vi "Measurement Logic.vi"(8 "error in":errorcluster, 9 "measurement configuration":T2={"Automation Test"=FALSE, "Power sequencing file path"="", "RFSG name"="5842_0", "RFSG port"="", "RFSG attenuation mode"=enum."Constant Attenuation", "RFSG external attenuation (dB)"=2.0, "RFSG s-parameters orientation"=enum."Port2 Towards DUT", "RFSG s2p file path"="", "RFmx name"="5842_0", "RFmx port"="", "RFmx attenuation mode"=enum."Constant Attenuation", "RFmx external attenuation (dB)"=1.2, "RFmx s-parameters orientation"=enum."Port2 Towards DUT", "RFmx s2p file path"="", "RFmx Center Frequency (Hz)"=10000000000.0, "RFmx Measurement Bandwidth (Hz)"=80000000.0, "RFmx Reference Level (dBm)"=10.0, "RFSG Generation IQ Rate (S/s)"=10000000000.0, "Pulse Acquisition Length (s)"=80000000.0, "Pulse Power Level (dBm)"=10.0, "Pulse Repetition Interval [PRI] (s)"=1250000000.0, "Pulse Width (s)"=0.001, "Number of Pulses per Burst"=0, "Measurement Offset"=0, "Window Start (%)"=2e-05, "Window Stop (%)"=20.0, "Window Step Size (%)"=0.0, "High Reference Level (%)"=10.0, "Width Reference Level (%)"=90.0, "Low Reference Level (%)"=10.0, "Selected Pulse Trace"=0, "Power sequencing file validity check"=FALSE} {"Width Reference Level (%)" format="%.2p"; "Window Stop (%)" format="%#_6p"; "Window Start (%)" format="%#_6p"; "Measurement Offset" format="%#_6p"; "Pulse Acquisition Length (s)" format="%.2f"; "Pulse Power Level (dBm)" format="%.6p"; "Number of Pulses per Burst" format="%.2f"; "Pulse Width (s)" format="%.3p"; "Pulse Repetition Interval [PRI] (s)" format="%.6p"; "RFSG Generation IQ Rate (S/s)" format="%.3p"; "RFmx Reference Level (dBm)" format="%.6p"; "RFmx Measurement Bandwidth (Hz)" format="%.3p"; "RFmx Center Frequency (Hz)" format="%.6p"; "RFmx external attenuation (dB)" format="%.2f"; "RFSG external attenuation (dB)" format="%.2f"}, 10 "measure call context in":refnum<class "Measure Call Context.lvclass">) -> (0 "error out":errorcluster, 1 "measurement results":T1, 2 "measure call context out":refnum<class "Measure Call Context.lvclass">)   [LabVIEW 2023, in "FPT Pulse Measurement.lvclass"]
doc: "Contains the core logic for executing the measurement."
uses:
  FPT Pulse Measurement.lvclass
  <vilib>/Plug-In SDKs/Measurements/Measure Call Context/Measure Call Context.lvclass
  Measurement Configuration.ctl
  Measurement Results.ctl
  <vilib>/Analysis/baseanly.llb/Mean (DBL).vi
  <extravilib>/ChannelInstances/Event Messenger-bool/Instantiate.vi
  FPT Pulse Measurement.lvclass/FPT Pulse Measurement.ctl
  <vilib>/Analysis/NI_AALBase.lvlib
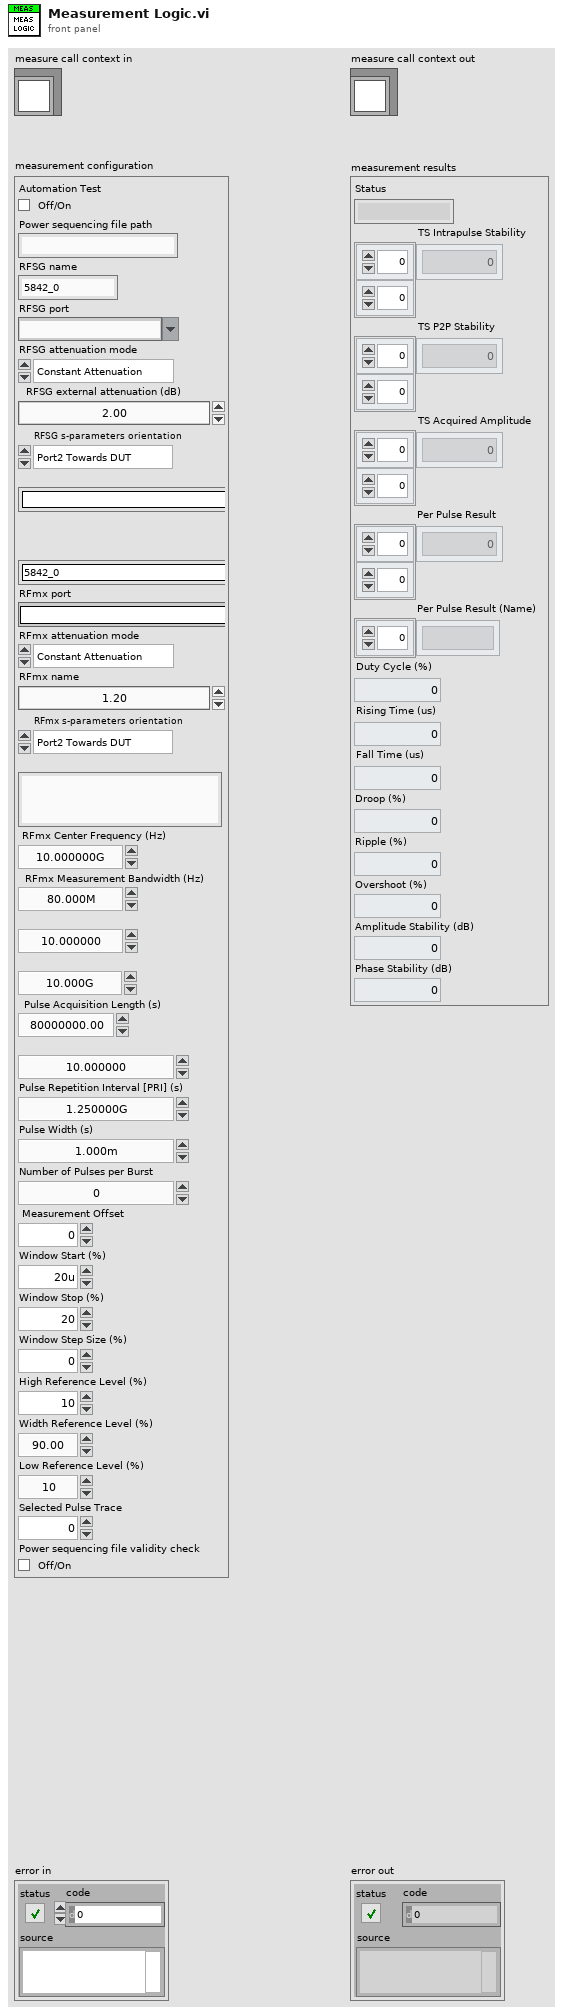
[diagram p1: front panel]
types:
  T1 = typedef "FPT Pulse Measurement.lvclass/Measurement Results.ctl" = cluster{"Status":string, "TS Intrapulse Stability":dbl[][], "TS P2P Stability":dbl[][], "TS Acquired Amplitude":dbl[][], "Per Pulse Result":dbl[][], "Per Pulse Result (Name)":string[], "Duty Cycle (%)":dbl, "Rising Time (us)":dbl, "Fall Time (us)":dbl, "Droop (%)":dbl, "Ripple (%)":dbl, "Overshoot (%)":dbl, "Amplitude Stability (dB)":dbl, "Phase Stability (dB)":dbl}
  T2 = typedef "FPT Pulse Measurement.lvclass/Measurement Configuration.ctl" = cluster{"Automation Test":bool, "Power sequencing file path":string, "RFSG name":string, "RFSG port":string, "RFSG attenuation mode":enum32{"<None>", "Constant Attenuation", "s2p File"}, "RFSG external attenuation (dB)":dbl, "RFSG s-parameters orientation":enum32{"Port1 Towards DUT", "Port2 Towards DUT"}, "RFSG s2p file path":string, "RFmx name":string, "RFmx port":string, "RFmx attenuation mode":enum32{"<None>", "Constant Attenuation", "s2p File"}, "RFmx external attenuation (dB)":dbl, "RFmx s-parameters orientation":enum32{"Port1 Towards DUT", "Port2 Towards DUT"}, "RFmx s2p file path":string, "RFmx Center Frequency (Hz)":dbl, "RFmx Measurement Bandwidth (Hz)":dbl, "RFmx Reference Level (dBm)":dbl, "RFSG Generation IQ Rate (S/s)":dbl, "Pulse Acquisition Length (s)":dbl, "Pulse Power Level (dBm)":dbl, "Pulse Repetition Interval [PRI] (s)":dbl, "Pulse Width (s)":dbl, "Number of Pulses per Burst":u32, "Measurement Offset":i32, "Window Start (%)":dbl, "Window Stop (%)":dbl, "Window Step Size (%)":dbl, "High Reference Level (%)":dbl, "Width Reference Level (%)":dbl, "Low Reference Level (%)":dbl, "Selected Pulse Trace":i32, "Power sequencing file validity check":bool}
  T3 = enum32{"Power On Dut", "De-embedding + Measurement", "Power Off Dut"}[]
  T4 = cluster{"measurement configuration":T2, "measurement results":T1, "CustomData":cluster{"Valid CSV":bool}}
  T5 = typedef "RFmx Config - Pulse.ctl" = cluster{"Center Frequency (Hz)":dbl, "Measurement Bandwidth (Hz)":dbl, "Reference Level (dBm)":dbl, "RFmx De-embedding":T6, "Acquisition Length (s)":dbl}
  T6 = typedef "RFmx Config.ctl" = cluster{"RFmx Name":refnum<k15>, "RFmx Port":string, "Attenuation":cluster{"Mode":enum32{"<None>", "Constant Attenuation", "s2p File"}, "Constant Attenuation":cluster{"RFmx External Attenuation (dB)":dbl}, "s2p File":cluster{"RFmx S-Parameters Orientation":i32, "RFmx Attenuation s2p Path Name":string, "RFmx Attenuation s2p File":path}}}
  T7 = typedef "RFSG Config - Pulse.ctl" = cluster{"RFSG De-embedding":T8, "Generation IQ Rate (S/s)":dbl}
  T8 = typedef "RFsg Config.ctl" = cluster{"RFSG Name":refnum<k15>, "RFSG Port":string, "Attenuation":cluster{"Mode":enum32{"<None>", "Constant Attenuation", "s2p File"}, "Contant Attenuation":cluster{"RFSG External Attenuation (dB)":dbl}, "s2p File":cluster{"RFSG S-parameters Orientation":i32, "RFSG Attenuation s2p Path Name":string, "RFSG s2p File Path":path}}}
  T9 = typedef "Test Config - Pulse.ctl" = cluster{"Pulse Configuration":cluster{"Power Level (dBm)":dbl, "Pulse Repetition Interval [PRI] (s)":dbl, "Pulse Width (s)":dbl, "Number of Pulses per Burst":u32}, "Pulse Stability":cluster{"Pulse Stability Meas Offset":i32, "Window Start (%)":dbl, "Window Stop (%)":dbl, "Window Step Size (%)":dbl, "Selected Pulse Trace":i32}, "Pulse Profile":cluster{"High Reference Level (%)":dbl, "Width Reference Level (%)":dbl, "Low Reference Level (%)":dbl}}
  T10 = typedef "Event Messenger-bool.lvlib/))Channel.ctl" = refnum<queue>
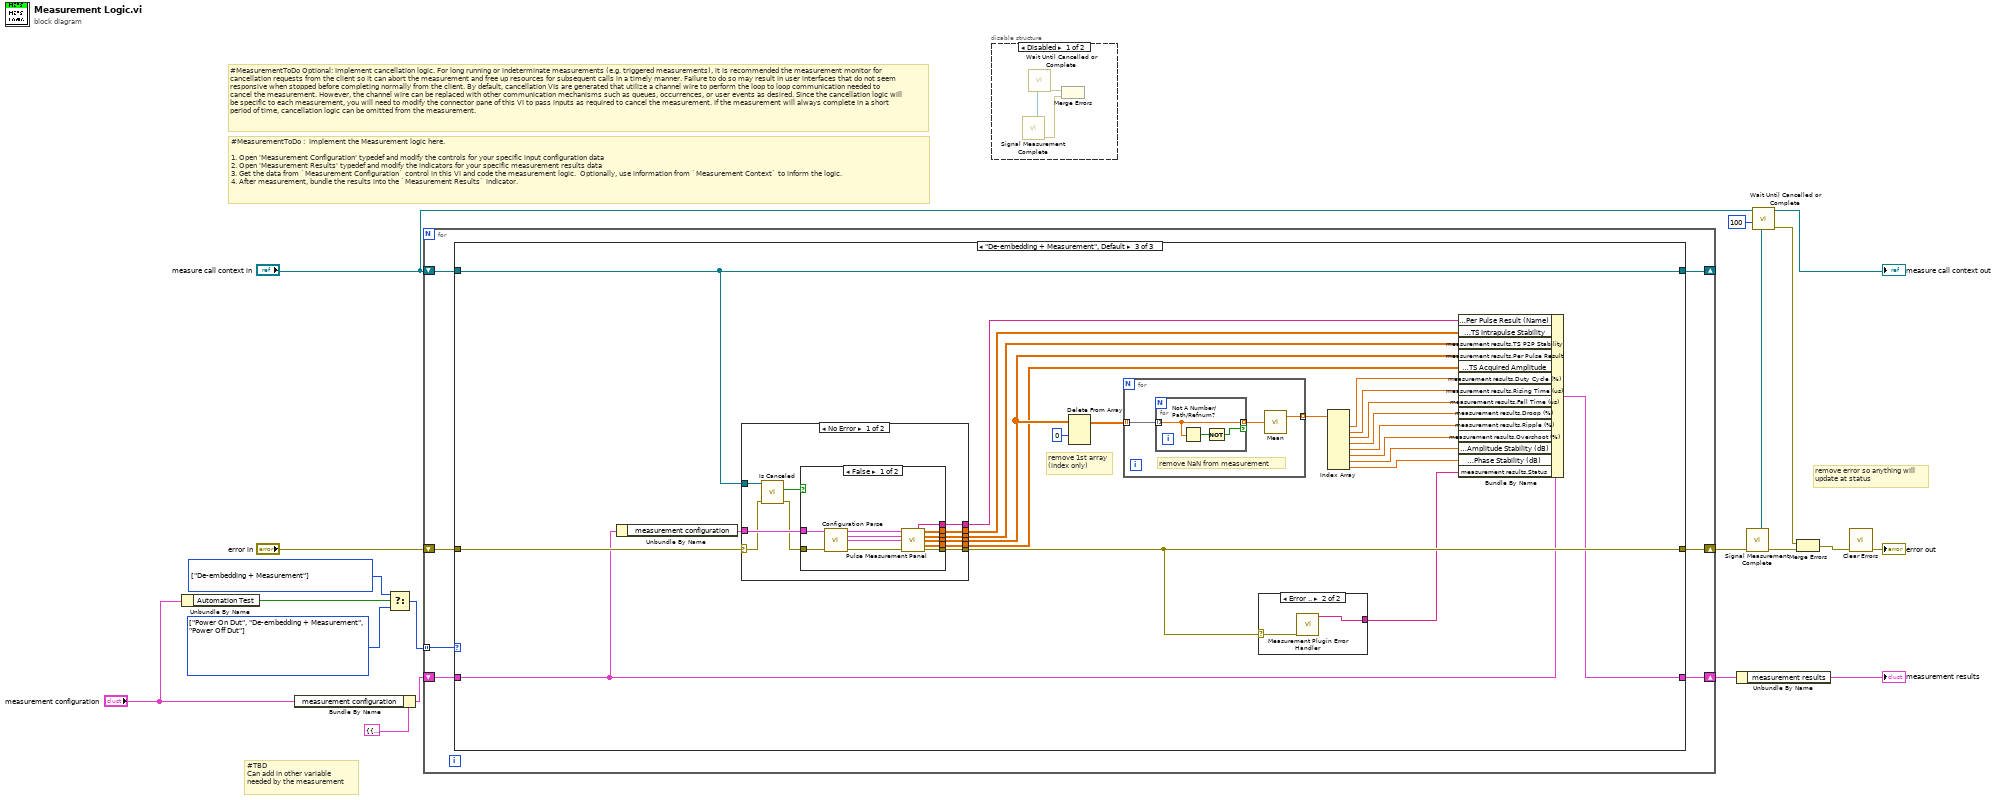
[diagram p0: block diagram]
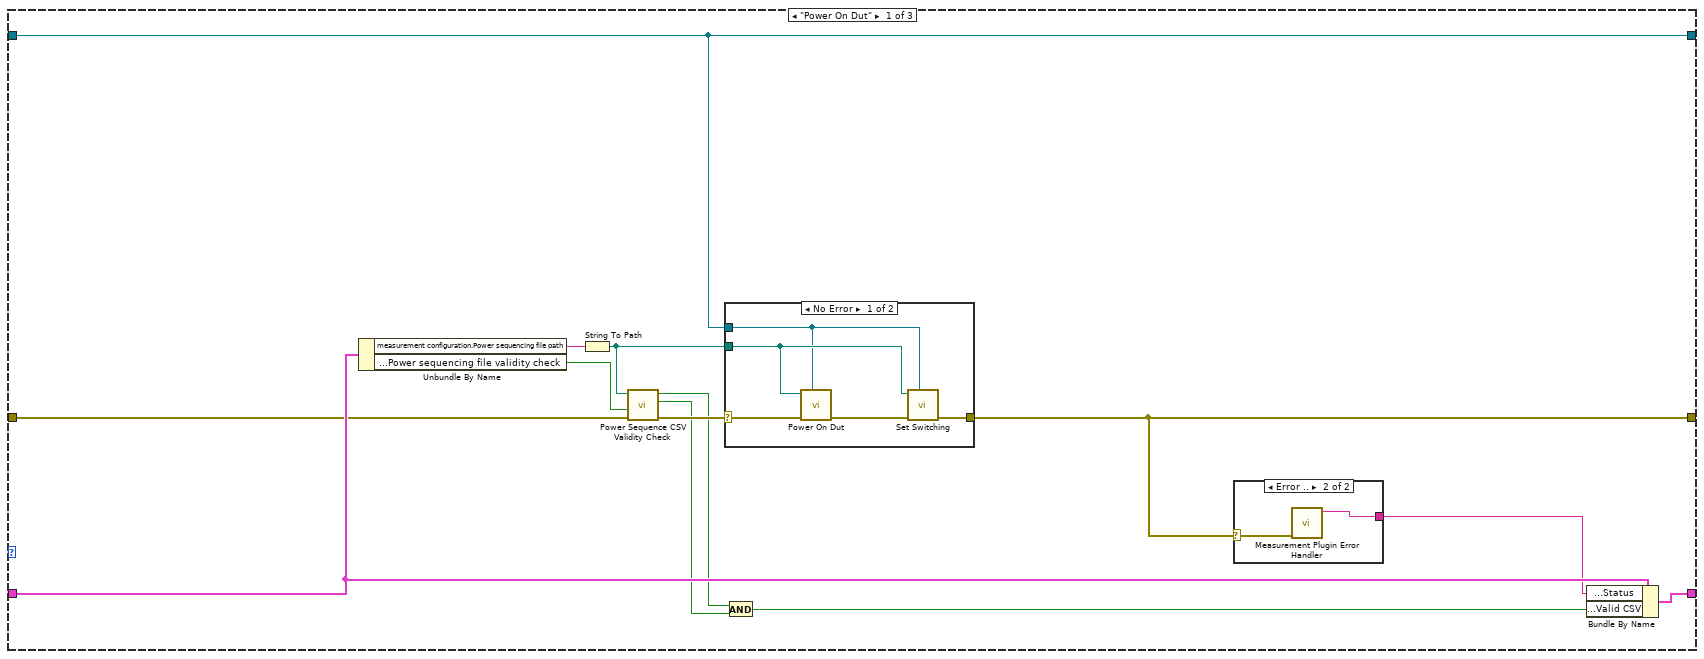
[diagram p2: hidden frame]
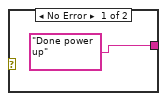
[diagram p4: hidden frame]
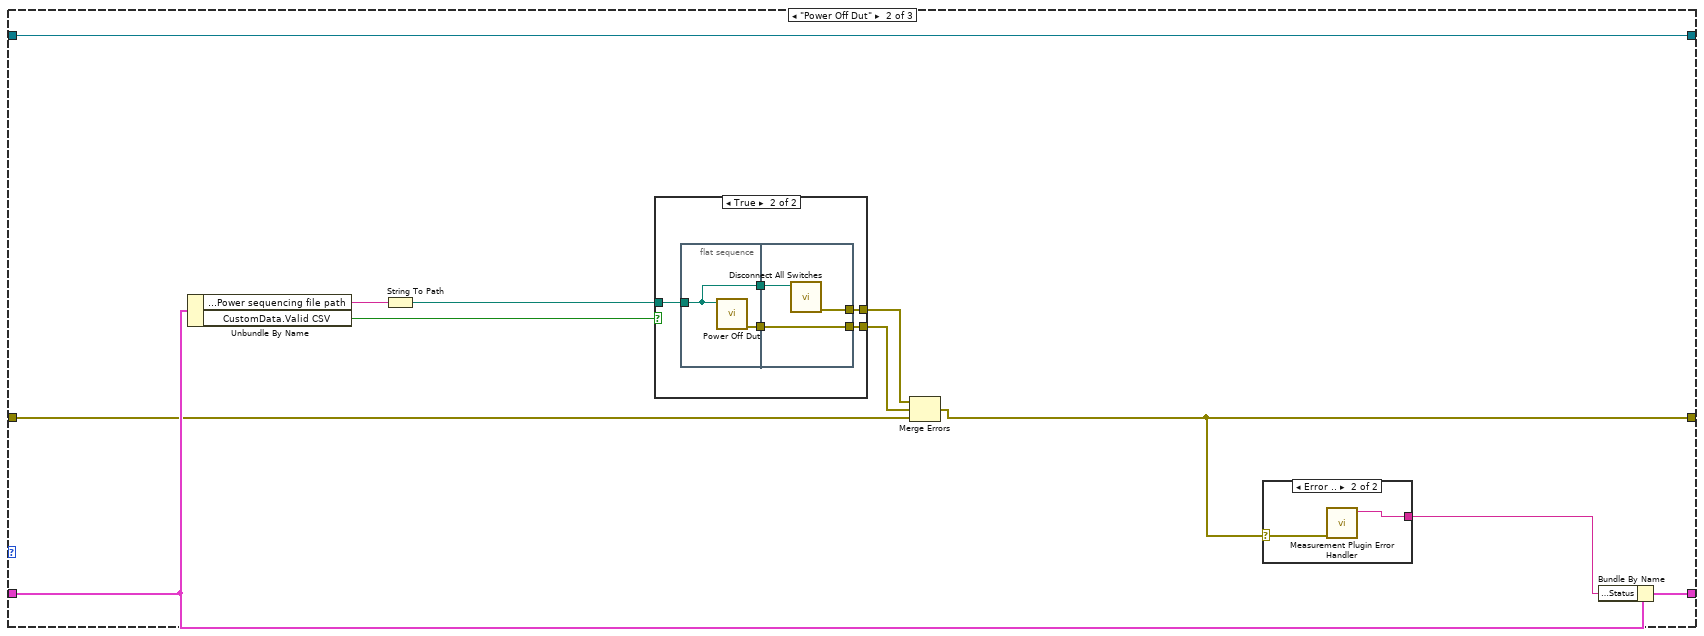
[diagram p5: hidden frame]
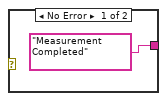
[diagram p7: hidden frame]
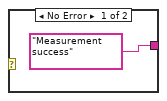
[diagram p8: hidden frame]
diagram:
  w9 = T3 [enum."De-embedding + Measurement"] items=["Power On Dut", "De-embedding + Measurement", "Power Off Dut"] ("t")
  w12 = T3 [enum."Power On Dut", enum."De-embedding + Measurement", enum."Power Off Dut"] items=["Power On Dut", "De-embedding + Measurement", "Power Off Dut"]
  # "remove error so anything will\nupdate at status"
  # "#TBD\nCan add in other variable\nneeded by the measurement"
  # "#MeasurementToDo Optional: Implement cancellation logic. For long running or indeterminate measurements (e.g. triggered measurements), it is recommended the measurement monitor for cancellation requests from the client so it can abort the measurement and free up resources for subsequent calls in a timely manner. Failure to do so may result in user interfaces that do not seem responsive when stopped before completing normally from the client. By default, cancellation VIs are generated that utilize a channel wire to perform the loop to loop communication needed to cancel the measurement. However, the channel wire can be replaced with other communication mechanisms such as queues, occurrences, or user events as desired. Since the cancellation logic will be specific to each measurement, you will need to modify the connector pane of this VI to pass inputs as required to cancel the measurement. If the measurement will always complete in a short period of time, cancellation logic can be omitted from the measurement."
  # "#MeasurementToDo :  Implement the Measurement logic here.\n\n1. Open 'Measurement Configuration' typedef and modify the controls for your specific input configuration data\n2. Open 'Measurement Results' typedef and modify the indicators for your specific measurement results data\n3. Get the data from `Measurement Configuration` control in this VI and code the measurement logic.  Optionally, use information from `Measurement Context` to inform the logic.\n4. After measurement, bundle the results into the `Measurement Results` indicator."
  n1 = Unbundle By Name("measurement configuration") -> ("Automation Test"=w11:bool)
  n2 = Bundle By Name(cluster=T4 {"measurement configuration"={"Automation Test"=FALSE, "Power sequencing file path"="", "RFSG name"="5842_0", "RFSG port"="", "RFSG attenuation mode"=enum."Constant Attenuation", "RFSG external attenuation (dB)"=2.0, "RFSG s-parameters orientation"=enum."Port2 Towards DUT", "RFSG s2p file path"="", "RFmx name"="5842_0", "RFmx port"="", "RFmx attenuation mode"=enum."Constant Attenuation", "RFmx external attenuation (dB)"=1.2, "RFmx s-parameters orientation"=enum."Port2 Towards DUT", "RFmx s2p file path"="", "RFmx Center Frequency (Hz)"=10000000000.0, "RFmx Measurement Bandwidth (Hz)"=80000000.0, "RFmx Reference Level (dBm)"=10.0, "RFSG Generation IQ Rate (S/s)"=10000000000.0, "Pulse Acquisition Length (s)"=80000000.0, "Pulse Power Level (dBm)"=10.0, "Pulse Repetition Interval [PRI] (s)"=1250000000.0, "Pulse Width (s)"=0.001, "Number of Pulses per Burst"=0, "Measurement Offset"=0, "Window Start (%)"=2e-05, "Window Stop (%)"=20.0, "Window Step Size (%)"=0.0, "High Reference Level (%)"=10.0, "Width Reference Level (%)"=90.0, "Low Reference Level (%)"=10.0, "Selected Pulse Trace"=0, "Power sequencing file validity check"=FALSE}, "measurement results"={"Status"="", "TS Intrapulse Stability"=[], "TS P2P Stability"=[], "TS Acquired Amplitude"=[], "Per Pulse Result"=[], "Per Pulse Result (Name)"=[], "Duty Cycle (%)"=0.0, "Rising Time (us)"=0.0, "Fall Time (us)"=0.0, "Droop (%)"=0.0, "Ripple (%)"=0.0, "Overshoot (%)"=0.0, "Amplitude Stability (dB)"=0.0, "Phase Stability (dB)"=0.0}, "CustomData"={"Valid CSV"=FALSE}}, "measurement configuration"="measurement configuration") -> (w17:T4)
  n3 = Select(t=w9, s=w11, f=w12) -> (s? t:f=w10:T3)
  n4 = for {
    shift-right: [w21] -> w7
    shift-left: "error in" -> [w26]
    shift-right: [w22] -> w16
    shift-left: w17 -> [w25]
    shift-right: [w23] -> _
    shift-left: "measure call context in" -> [w24]
    tunnel: w10 -> [w20] mode=indexing
    n5 = case shown="\"De-embedding + Measurement\", Default" w20 {
      tunnel: w26 -> [w33 w54 w76]
      tunnel: w25 -> [w39 w55 w75]
      tunnel: w24 -> [w34 w58 w74]
      tunnel: [w35 w53 w95] -> w21
      tunnel: [w34 w58 w74] -> w23
      tunnel: [w37 w56 w94] -> w22
      frame "Power On Dut" {
        n6 = Unbundle By Name(w39) -> ("measurement configuration.Power sequencing file path"=w36:string, "measurement configuration.Power sequencing file validity check"=w32:bool)
        n7 = String To Path(string=w36) -> (path=w31:path)
        n8 = call "Power Sequence CSV Validity Check.vi"("error in"=w33, "Enable Validity Check?"=w32, "File Path"=w31) -> ("error out"=w30:errorcluster, "Valid Execution Order"=w28:bool, "All Instruments Available"=w29:bool)  [unwired: 5 in, 1 out]
        n9 = case shown="No Error" w30 {
          selector: w30 -> [w40 w45]
          tunnel: [w44 w45] -> w35
          tunnel: w31 -> [w42 _]
          tunnel: w34 -> [w41 _]
          frame No Error {
            n10 = call "Power On Dut.vi"("measure call context in"=w41, "error in"=w40, "Power sequencing file path"=w42) -> ("error out"=w43:errorcluster)  [unwired: 7 in, 1 out]
            n11 = call "Set Switching.vi"("measure call context in"=w41, "error in"=w43, "File Path"=w42) -> ("error out"=w44:errorcluster)  [unwired: 7 in, 1 out]
          }
          frame Error {
          }
        }
        n12 = And(x=w29, y=w28) -> (x .and. y?=w27:bool)
        n13 = case shown="Error .." w35 {
          selector: w35 -> [_ w48]
          tunnel: ["Done power up" w47] -> w38
          frame No Error {
          }
          frame Error {
            n14 = call "Measurement Plugin Error Handler.vi"("error in"=w48) -> ("Status Message (Error)"=w47:string)  [unwired: 9 in, 1 out]
          }
        }
        n15 = Bundle By Name(cluster=w39, "measurement results.Status"=w38, "CustomData.Valid CSV"=w27) -> (w37:T4)
      }
      frame "Power Off Dut" {
        n16 = Unbundle By Name(w55) -> ("measurement configuration.Power sequencing file path"=w59:string, "CustomData.Valid CSV"=w49:bool)
        n17 = String To Path(string=w59) -> (path=w52:path)
        n18 = case shown="True" w49 {
          tunnel: w52 -> [_ w62]
          tunnel: [_ w61] -> w51
          tunnel: [_ w60] -> w50
          frame False {
          }
          frame True {
            n19 = flat-sequence {
              tunnel: w62 -> [w65]
              tunnel: [w66] -> w64
              tunnel: [w65] -> w63
              tunnel: [w69] -> w61
              tunnel: w64 -> [w69]
              tunnel: [w68] -> w60
              tunnel: w63 -> [w67]
              frame #0 {
                n20 = call "Power Off Dut.vi"("Power Sequencing File Path"=w65) -> ("error out"=w66:errorcluster)  [unwired: 10 in]
              }
              frame #1 {
                n21 = call "Disconnect All Switches.vi"("File Path"=w67) -> ("error out"=w68:errorcluster)  [unwired: 10 in]
              }
            }
          }
        }
        n22 = Merge Errors(w50, w51, w54) -> (w53:errorcluster)
        n23 = case shown="Error .." w53 {
          selector: w53 -> [_ w72]
          tunnel: ["Measurement Completed" w71] -> w57
          frame No Error {
          }
          frame Error {
            n24 = call "Measurement Plugin Error Handler.vi"("error in"=w72) -> ("Status Message (Error)"=w71:string)  [unwired: 9 in, 1 out]
          }
        }
        n25 = Bundle By Name(cluster=w55, "measurement results.Status"=w57) -> (w56:T4)
      }
      frame "De-embedding + Measurement", Default {
        # "remove 1st array\n(index only)"
        n26 = Unbundle By Name(w75) -> ("measurement configuration"=w73:T2)
        n27 = case shown="No Error" w76 {
          selector: w76 -> [w100 w123]
          tunnel: [w109 w123] -> w95
          tunnel: [w108 _] -> w93
          tunnel: [w107 _] -> w92
          tunnel: [w106 _] -> w91
          tunnel: [w105 _] -> w86
          tunnel: [w104 _] -> w77
          tunnel: w73 -> [w103 _]
          tunnel: w74 -> [w99 _]
          frame No Error {
            n28 = call <vilib>:"Is Canceled.vi"("error in"=w100, "measure call context in"=w99) -> ("error out"=w101:errorcluster, "is canceled?"=w102:bool)  [unwired: 7 in, 1 out]
            n29 = case shown="False" w102 {
              tunnel: [w121 w122] -> w109
              tunnel: [w116 _] -> w108
              tunnel: [w115 _] -> w107
              tunnel: [w114 _] -> w106
              tunnel: [w113 _] -> w105
              tunnel: [w112 _] -> w104
              tunnel: w103 -> [w111 _]
              tunnel: w101 -> [w110 w122]
              frame False {
                n30 = call "Configuration Parse.vi"("Measurement Configuration"=w111, "error in"=w110) -> ("RFmx Settings"=w119:T5, "RFSG settings"=w118:T7, "Test Configuration"=w117:T9, "error out"=w120:errorcluster)  [unwired: 10 in]
                n31 = call "Pulse Measurement Panel.vi"("RFmx Settings"=w119, "RFSG settings"=w118, "Test Configuration"=w117, "error in"=w120) -> ("Per Pulse Results (Header Name)"=w113:string[], "TS Intrapulse Stability"=w115:dbl[][], "TS P2P Stability"=w116:dbl[][], "Per Pulse Results (for MP)"=w114:dbl[][], "TS Acquired Amplitude"=w112:dbl[][], "error out"=w121:errorcluster)  [unwired: 6 in]
              }
              frame True {
              }
            }
          }
          frame Error {
          }
        }
        n32 = Delete From Array(array=w91, index (row)=0) -> (array with subset deleted=w89:dbl[][])  [unwired: 2 in, 1 out]
        n33 = for {
          tunnel: w89 -> [w125] mode=indexing
          tunnel: [w126] -> w87 mode=indexing
          # "remove NaN from measurement"
          n34 = for {
            tunnel: w125 -> [w128] mode=indexing
            tunnel: [w128] -> w124 mode=indexing if=w127
            n35 = Not A Number/Path/Refnum?(number/path/refnum=w128) -> (NaN/Path/Refnum?=w129:bool)
            n36 = Not(x=w129) -> (.not. x?=w127:bool)
          }
          n37 = call-poly <vilib>:"Mean.vi"("X"=w124) -> ("mean"=w126:dbl)  [unwired: 1 out]
        }
        n38 = case shown="Error .." w95 {
          selector: w95 -> [_ w98]
          tunnel: ["Measurement success" w97] -> w88
          frame No Error {
          }
          frame Error {
            n39 = call "Measurement Plugin Error Handler.vi"("error in"=w98) -> ("Status Message (Error)"=w97:string)  [unwired: 9 in, 1 out]
          }
        }
        n40 = Index Array(array=w87) -> (element #1=w78:dbl, element #2=w85:dbl, element #3=w84:dbl, element #4=w83:dbl, element #5=w82:dbl, element #6=w81:dbl, element #7=w80:dbl, element #8=w79:dbl)  [unwired: 8 in]
        n41 = Bundle By Name(cluster=w75, "measurement results.Per Pulse Result (Name)"=w86, "measurement results.TS Intrapulse Stability"=w92, "measurement results.TS P2P Stability"=w93, "measurement results.Per Pulse Result"=w91, "measurement results.TS Acquired Amplitude"=w77, "measurement results.Duty Cycle (%)"=w78, "measurement results.Rising Time (us)"=w85, "measurement results.Fall Time (us)"=w84, "measurement results.Droop (%)"=w83, "measurement results.Ripple (%)"=w82, "measurement results.Overshoot (%)"=w81, "measurement results.Amplitude Stability (dB)"=w80, "measurement results.Phase Stability (dB)"=w79, "measurement results.Status"=w88) -> (w94:T4)
      }
    }
  }
  n42 = disable-structure shown="Disabled" {
    frame Disabled {
      n43 = call "Signal Measurement Complete.vi"() -> ("error out"=w131:errorcluster, "done channel"=w132:T10)  [unwired: 10 in]
      n44 = call "Wait Until Cancelled or Complete.vi"("done channel"=w132) -> ("error out"=w130:errorcluster)  [unwired: 9 in, 1 out]
      n45 = Merge Errors(w130, w131) -> ()  [unwired: 1 out]
    }
    frame Enabled {
    }
  }
  n46 = Unbundle By Name(w16) -> ("measurement results"=→"measurement results":T1)
  n47 = call "Signal Measurement Complete.vi"("error in (no error)"=w7) -> ("error out"=w8:errorcluster, "done channel"=w4:T10)  [unwired: 9 in]
  n48 = call "Wait Until Cancelled or Complete.vi"("done channel"=w4, "ms polling interval"=100, "measure call context in"="measure call context in") -> ("error out"=w2:errorcluster, "measure call context out"=→"measure call context out":refnum<class "Measure Call Context.lvclass">)  [unwired: 7 in]
  n49 = Merge Errors(w2, w8) -> (w3:errorcluster)
  n50 = call <vilib>:"Clear Errors.vi"("error in (no error)"=w3) -> ("error out"=→"error out":errorcluster)  [unwired: 5 in, 1 out]
